vi "Set configuration chain.vi"(8 "error in (no error)":errorcluster, 9 "class names":string[](array[string]), 10 "configuration":variant[](array[variant]), 11 "ImageStack in":refnum<class "ImageStack.lvclass">) -> (0 "error out":errorcluster, 3 "ImageStack out":refnum<class "ImageStack.lvclass">)   [LabVIEW 2012, in "ImageStack.lvclass"]
uses:
  ImageStack.lvclass
  <vilib>/Distrio/Murmex/Murmex/Murmex.lvclass
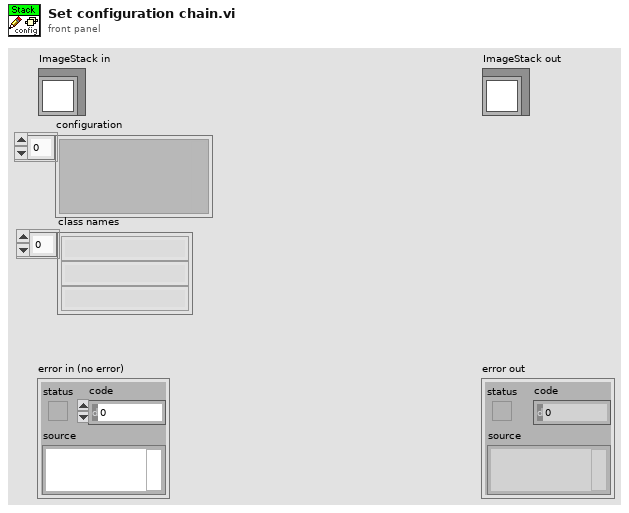
[diagram p1: front panel]
types:
  T1 = typedef "ImageStack.lvclass/configuration_cluster.ctl" = cluster{"Camera component name":string, "Stages component name":string, "AOTF component name":string}
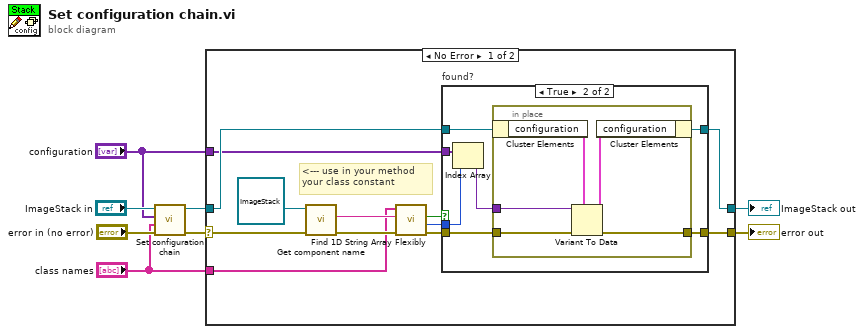
[diagram p0: block diagram]
diagram:
  n1 = call-parent "Set configuration chain.vi"("error in (no error)"="error in (no error)", "class names"="class names", "configuration"="configuration", "Murmex in"="ImageStack in") -> ("error out"=w6:errorcluster, "Murmex out"=w3:refnum<class "ImageStack.lvclass">)  [unwired: 6 in]
  n2 = case shown="No Error" w6 {
    selector: w6 -> [w15 w36]
    tunnel: [w10 w36] -> w5
    tunnel: [w11 w35] -> w4
    tunnel: w3 -> [w14 w35]
    tunnel: "configuration" -> [w13 _]
    tunnel: "class names" -> [w12 _]
    frame No Error {
      # "<--- use in your method\nyour class constant"
      n3 = call <vilib>:"Get component name.vi"("error in (no error)"=w15, "Murmex in"=refnum<class "ImageStack.lvclass"> refnum ("ImageStack in")) -> ("error out"=w16:errorcluster, "component name"=w18:string)  [unwired: 7 in, 1 out]
      n4 = call <vilib>:"Find 1D String Array Flexibly.vi"("error in (no error)"=w16, "element"=w18, "array"=w12) -> ("error out"=w17:errorcluster, "index of element"=w19:i32, "found?"=w20:bool)  [unwired: 6 in]
      n5 = case "found?" shown="True" w20 {
        tunnel: w13 -> [_ w29]
        tunnel: w14 -> [w22 w27]
        tunnel: [w22 w26] -> w11
        tunnel: [w21 w25] -> w10
        tunnel: w17 -> [w21 w24]
        tunnel: w19 -> [_ w23]
        frame False {
        }
        frame True {
          n6 = Index Array(array=w29, index=w23) -> (element=w28:variant)
          n7 = in-place {
            in-place-border: w28 -> [w34]
            in-place-border: w24 -> [w32]
            in-place-border: [w30] -> w25
            n8 = in-place-cluster #1(w27) -> ("configuration"=w33:T1)
            n9 = Variant To Data(error in=w32, type=w33, Variant=w34) -> (data=w31:T1, error out=w30:errorcluster)
            n10 = in-place-cluster #1("configuration"=w31) -> (w26:refnum<class "ImageStack.lvclass">)
          }
        }
      }
    }
    frame Error {
    }
  }
  "error out" <- w5
  "ImageStack out" <- w4
